vi "H5Ldelete.vi"(6 "lapl_id":T1, 8 "error in (no error)":errorcluster, 10 "Name":string, 11 "Location Ref":T1) -> (0 "error out":errorcluster, 3 "Location Ref out":T1)   [LabVIEW 2017]
doc: "Removes a link from a group."
uses:
  <vilib>/UPVI/lvhdf5/library.llb/HDF5 Ref.ctl
  <vilib>/UPVI/lvhdf5/hdf5.dll
panel:
  # "LVHDF5 Toolkit\nCopyright (c) 2005-2013 by Jason D. Sommerville\nCopyright (c) 2014-2015 by UPVI, LLC.\n\nThis use and distribution of this file is governed by the terms found in \nLICENSE.txt distributed with this toolkit and installed at\n <user.lib>\\_lvhdf5\\LICENSE.txt"
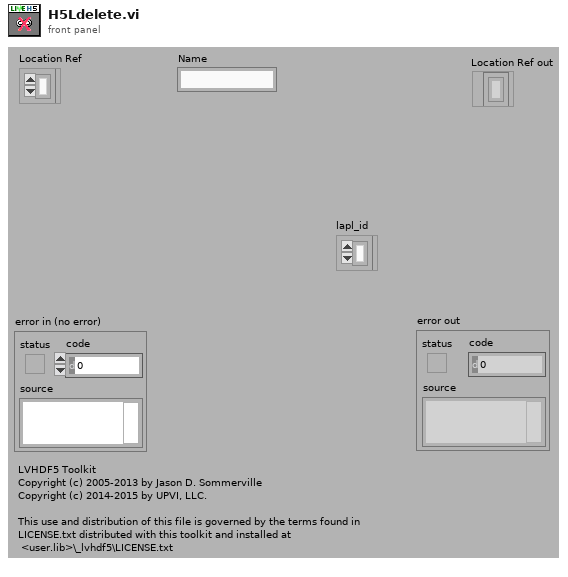
[diagram p1: front panel]
types:
  T1 = typedef "HDF5 Ref.ctl" = refnum<k1>
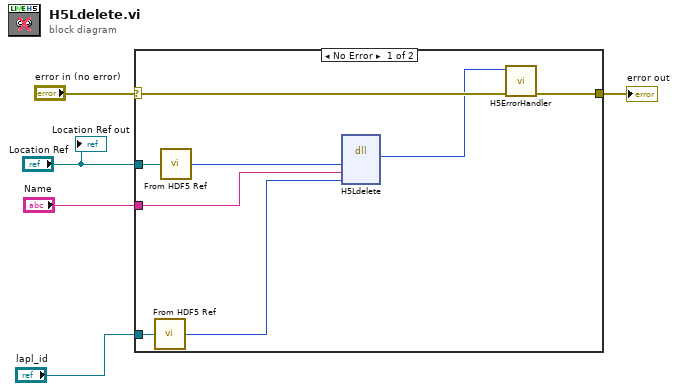
[diagram p0: block diagram]
diagram:
  n1 = case shown="No Error" "error in (no error)" {
    selector: "error in (no error)" -> [w13 w14]
    tunnel: [w12 w14] -> w4
    tunnel: "Location Ref" -> [w11 _]
    tunnel: "Name" -> [w7 _]
    tunnel: "lapl_id" -> [w6 _]
    frame No Error {
      n2 = call <vilib>:"From HDF5 Ref.vi"("HDF5 Ref"=w6) -> ("I32"=w10:i32)
      n3 = call <vilib>:"From HDF5 Ref.vi"("HDF5 Ref"=w11) -> ("I32"=w9:i32)
      n4 = dll-call lib="C:/Program Files/National Instruments/LabVIEW 2017/vi.lib/UPVI/lvhdf5/hdf5.dll" fn="H5Ldelete"("loc_id"=w9, "name"=w7, "lapl_id"=w10) -> ("return type"=w8:i32)  [unwired: 6 in, 2 out]
      n5 = call <vilib>:"H5ErrorHandler.vi"("error in (no error)"=w13, "herr_t"=w8) -> ("error out"=w12:errorcluster)  [unwired: 3 in, 4 out]
    }
    frame Error {
    }
  }
  "error out" <- w4
  "Location Ref out" <- "Location Ref"
